vi "Demo- Create and Update Feature Studio in new document.vi"() -> ()   [LabVIEW 2019]
panel:
  in  "FeatureScript":string
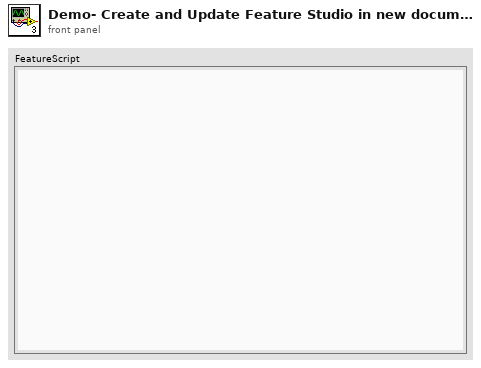
[diagram p1: front panel]
types:
  T1 = typedef "Cluster.ctl" = cluster{"Date":string, "On-Nonce":string, "eid":string, "wid":string, "did":string, "name":string, "method":string, "Accept":string, "User-Agent":string, "Content-Type":string, "stack":string, "headers":string[], "payload":string, "ctype":string, "path":string, "Authorization":string, "secret_key":string, "access_key":string}
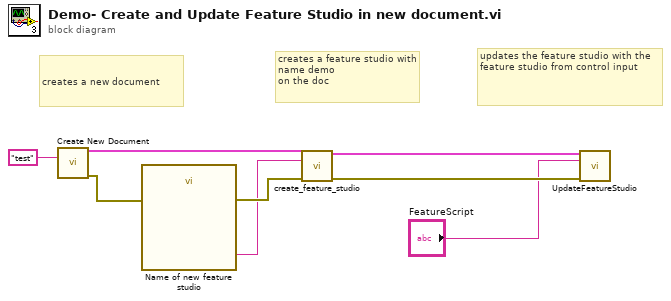
[diagram p0: block diagram]
diagram:
  # "creates a new document"
  # "updates the feature studio with the feature studio from control input"
  # "creates a feature studio with name demo\non the doc"
  n1 = call "Create New Document.vi"("Name In"="test") -> ("Device Out"=w6:T1, "error out"=w5:errorcluster)  [unwired: 12 in, 1 out]
  n2 = call "Name of new feature studio"("error in (no error)"=w5) -> ("Name"=w3:string, "error out"=w4:errorcluster)  [unwired: 16 in, 1 out]
  n3 = call "create_feature_studio.vi"("Device In"=w6, "New Feature Studio Name"=w3, "error in"=w4) -> ("Device Out"=w8:T1, "error out"=w7:errorcluster)  [unwired: 10 in, 1 out]
  n4 = call "UpdateFeatureStudio.vi"("Device In"=w8, "FeatureScript"="FeatureScript", "error in"=w7) -> ()  [unwired: 10 in, 3 out]
